vi "VolumeCoordinate.vi"(10 "PointNum":u32, 11 "Scan Settings":T1) -> (2 "RepNum":u32, 3 "Point":cluster{"X":i32, "Y":i32, "Z":i32})   [LabVIEW 2011]
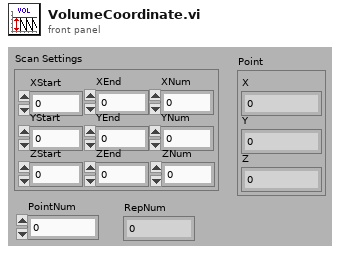
[diagram p1: front panel]
types:
  T1 = cluster{"XStart":i32, "XEnd":i32, "XNum":i32, "YStart":i32, "YEnd":i32, "YNum":i32, "ZStart":i32, "ZEnd":i32, "ZNum":i32}
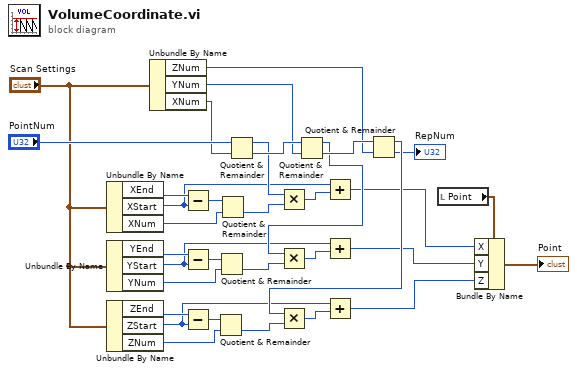
[diagram p0: block diagram]
diagram:
  n1 = Unbundle By Name("Scan Settings") -> ("XEnd"=w23:i32, "XStart"=w4:i32, "XNum"=w6:i32)
  n2 = Unbundle By Name("Scan Settings") -> ("YEnd"=w21:i32, "YStart"=w3:i32, "YNum"=w9:i32)
  n3 = Unbundle By Name("Scan Settings") -> ("ZEnd"=w17:i32, "ZStart"=w2:i32, "ZNum"=w12:i32)
  n4 = Unbundle By Name("Scan Settings") -> ("ZNum"=w29:i32, "YNum"=w31:i32, "XNum"=w33:i32)
  n5 = Subtract(x=w23, y=w4) -> (x-y=w7:i32)
  n6 = Subtract(x=w21, y=w3) -> (x-y=w10:i32)
  n7 = Subtract(x=w17, y=w2) -> (x-y=w13:i32)
  n8 = Quotient & Remainder(x=w13, y=w12) -> (floor(x/y)=w11:i32)  [unwired: 1 out]
  n9 = Quotient & Remainder(x=w10, y=w9) -> (floor(x/y)=w8:i32)  [unwired: 1 out]
  n10 = Quotient & Remainder(x=w7, y=w6) -> (floor(x/y)=w5:i32)  [unwired: 1 out]
  n11 = Quotient & Remainder(x="PointNum", y=w33) -> (x-y*floor(x/y)=w25:u32, floor(x/y)=w32:u32)
  n12 = Multiply(x=w25, y=w5) -> (x*y=w24:u32)
  n13 = Quotient & Remainder(x=w32, y=w31) -> (x-y*floor(x/y)=w20:u32, floor(x/y)=w30:u32)
  n14 = Multiply(x=w20, y=w8) -> (x*y=w22:u32)
  n15 = Add(x=w4, y=w24) -> (x+y=w16:u32)
  n16 = Add(x=w3, y=w22) -> (x+y=w15:u32)
  n17 = Quotient & Remainder(x=w30, y=w29) -> (x-y*floor(x/y)=w18:u32, floor(x/y)=→"RepNum":u32)
  n18 = Multiply(x=w18, y=w11) -> (x*y=w19:u32)
  n19 = Add(x=w2, y=w19) -> (x+y=w14:u32)
  n20 = local read "Point"() -> (w28:cluster{"X":i32, "Y":i32, "Z":i32})
  n21 = Bundle By Name(cluster=w28, "X"=w16, "Y"=w15, "Z"=w14) -> (→"Point":cluster{"X":i32, "Y":i32, "Z":i32})
